vi "RotatePolarization.vi"(9 "End Pos":dbl, 10 "curr pos":dbl) -> (2 "Pos out":dbl)   [LabVIEW 2015]
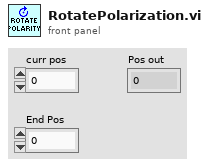
[diagram p1: front panel]
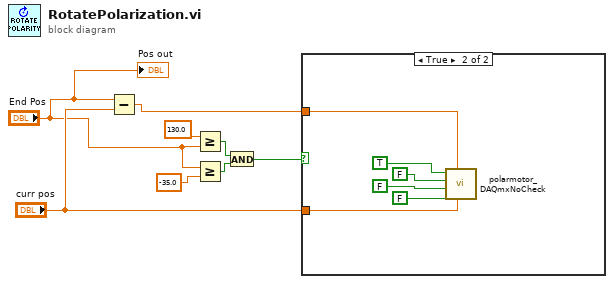
[diagram p0: block diagram]
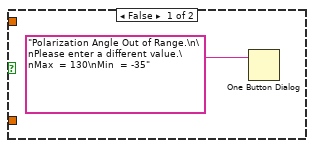
[diagram p2: hidden frame]
diagram:
  n1 = Subtract(x="End Pos", y="curr pos") -> (x-y=w2:dbl)
  n2 = Greater Or Equal?(x=130.0, y="End Pos") -> (x >= y?=w5:bool)
  n3 = Greater Or Equal?(x="End Pos", y=-35.0) -> (x >= y?=w6:bool)
  n4 = And(x=w5, y=w6) -> (x .and. y?=w4:bool)
  n5 = case shown="True" w4 {
    tunnel: w2 -> [_ w11]
    tunnel: "curr pos" -> [_ w10]
    frame False {
      n6 = One Button Dialog(message="Polarization Angle Out of Range.\n\nPlease enter a different value.\nMax  = 130\nMin  = -35") -> ()  [unwired: 1 in, 1 out]
    }
    frame True {
      n7 = call "polarmotor_DAQmxNoCheck.vi"("Position (Deg) 2"=w10, "Num Degrees"=w11, "Free"=FALSE, "Free2"=FALSE, "Speed"=FALSE, "C-on"=TRUE) -> ()  [unwired: 4 in, 2 out]
    }
  }
  "Pos out" <- "End Pos"
